vi "CMD_Reset.vi"(1 "Line":string) -> (0 "Done":bool)   [LabVIEW 2015]
panel:
  in  "Parameters":i32[](array[numeric])=[0, 1, 0]
  in  "Subcommands":string[](array[string])=["gyro", "gyro", "encoders"]
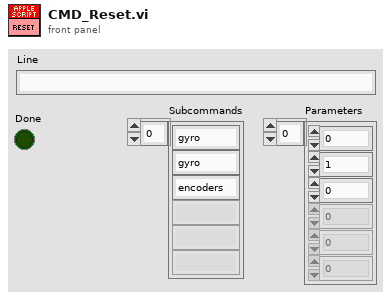
[diagram p1: front panel]
types:
  T1 = typedef "WPI_EncoderDevRef.ctl" = cluster{"DevStatus":errorcluster, "EncoderIndex":T2, "CounterIndex":T3, "DistancePerCount":dbl, "Decoding Type":T4}
  T2 = typedef "FPGA_EncoderIdx.ctl" = enum8{"Enc 0", "Enc 1", "Enc 2", "Enc 3", "Enc 4", "Enc 5", "Enc 6", "Enc 7", "Invalid"}
  T3 = typedef "FPGA_CounterCtrSystemIndex.ctl" = enum8{"Ctr 0", "Ctr 1", "Ctr 2", "Ctr 3", "Ctr 4", "Ctr 5", "Ctr 6", "Ctr 7", "Invalid"}
  T4 = typedef "WPI_EncoderType.ctl" = enum16{"1x", "2x", "4x"}
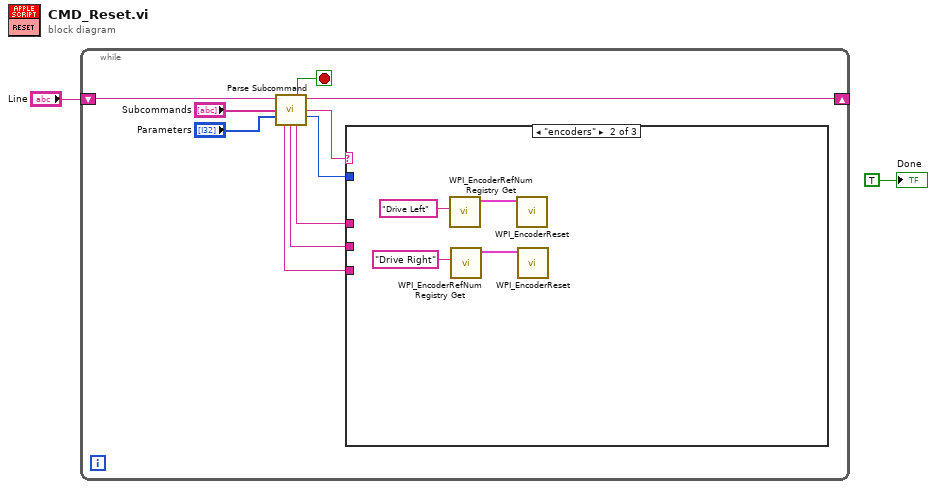
[diagram p0: block diagram]
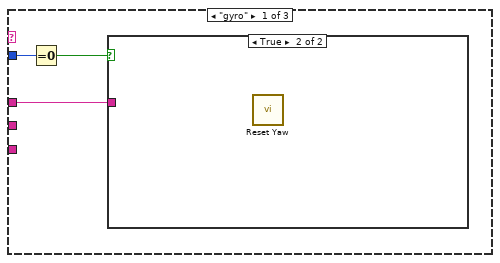
[diagram p2: hidden frame]
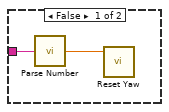
[diagram p3: hidden frame]
diagram:
  n1 = while {
    shift-right: [w9] -> _
    shift-left: "Line" -> [w12]
    stop <- w8 stop-if-true
    n2 = call "Parse Subcommand.vi"("Text In"=w12, "Subcommands"="Subcommands", "Parameters"="Parameters") -> ("Done"=w8:bool, "Text Out"=w9:string, "Subcommand"=w7:string, "# of Parameters"=w6:i32, "Parameter 3"=w3:string, "Parameter 2"=w4:string, "Parameter 1"=w5:string)  [unwired: 6 in]
    n3 = case shown="\"encoders\"" w7 {
      tunnel: w6 -> [w15 _ _]
      tunnel: w5 -> [w13 _ _]
      tunnel: w4 -> [_ _ _]
      tunnel: w3 -> [_ _ _]
      frame "gyro" {
        n4 = Equal To 0?(x=w15) -> (x = 0?=w14:bool)
        n5 = case shown="True" w14 {
          tunnel: w13 -> [w17 _]
          frame False {
            n6 = call "Parse Number.vi"("String"=w17) -> ("Number"=w16:dbl)
            n7 = call "Reset Yaw.vi"("To"=w16) -> ()  [unwired: 11 in]
          }
          frame True {
            n8 = call "Reset Yaw.vi"() -> ()  [unwired: 12 in]
          }
        }
      }
      frame "encoders" {
        n9 = call <vilib>:"WPI_EncoderRefNum Registry Get.vi"("refnum name"="Drive Left") -> ("EncoderDevRef"=w19:T1)  [unwired: 9 in, 1 out]
        n10 = call <vilib>:"WPI_EncoderRefNum Registry Get.vi"("refnum name"="Drive Right") -> ("EncoderDevRef"=w20:T1)  [unwired: 9 in, 1 out]
        n11 = call <vilib>:"WPI_EncoderReset.vi"("EncoderDevRef"=w19) -> ()  [unwired: 9 in, 2 out]
        n12 = call <vilib>:"WPI_EncoderReset.vi"("EncoderDevRef"=w20) -> ()  [unwired: 9 in, 2 out]
      }
      frame Default {
        # "If subcommand not recognized"
      }
    }
  }
  "Done" <- TRUE
